vi "Structs.vi"() -> ()   [LabVIEW 2019]
uses:
  Cluster2.ctl
  Cluster1.ctl
panel:
  in  "Cluster":T1
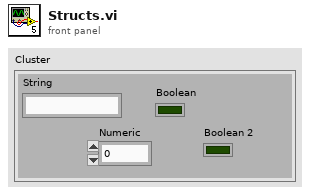
[diagram p1: front panel]
types:
  T1 = typedef "Cluster2.ctl" = cluster{"String":T2, "Boolean":bool, "Numeric":dbl, "Boolean 2":bool}
  T2 = typedef "Cluster1.ctl" = string
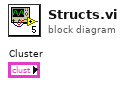
[diagram p0: block diagram]
diagram:
